vi "Insert Walls in Map.vi"(0 "Map":T1, 1 "Grid size":dbl=0.1, 2 "# safety grids":i32, 3 "Walls":cluster{"Y":dbl, "X":dbl}[](array[cluster])) -> (5 "Updated Map":T1)   [LabVIEW 2009]
uses:
  <vilib>/Analysis/Matrix/Datatypes/RealMatrix.ctl
  <vilib>/Analysis/Matrix/NI_Matrix.lvlib
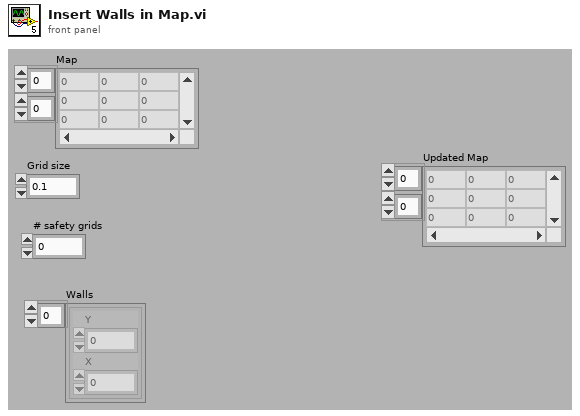
[diagram p1: front panel]
types:
  T1 = typedef "NI_Matrix.lvlib/RealMatrix.ctl" = dbl[][]
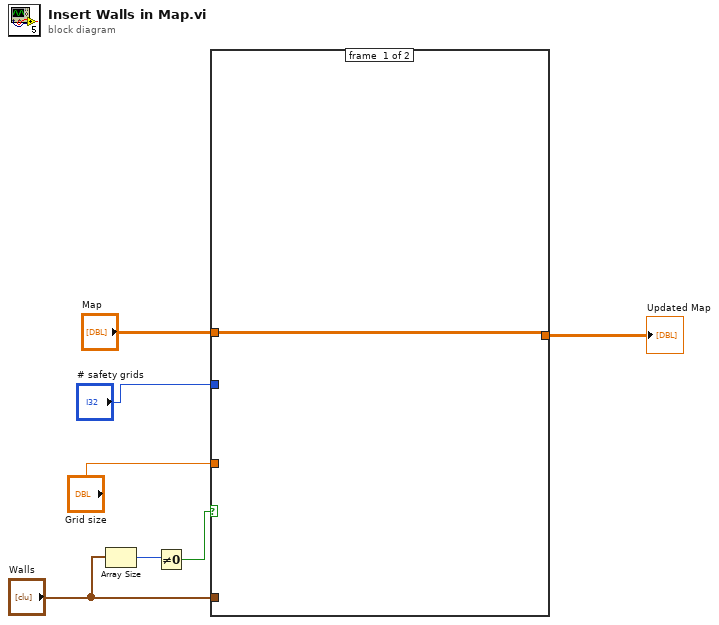
[diagram p0: block diagram]
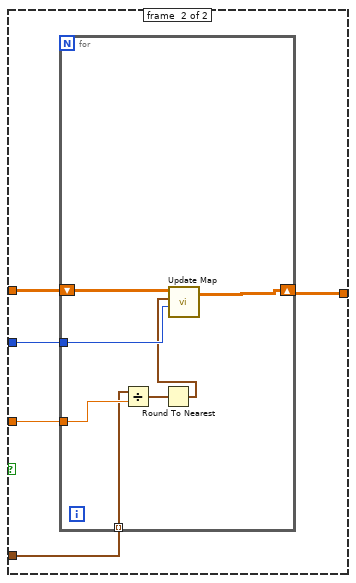
[diagram p2: hidden frame]
diagram:
  n1 = Array Size(array="Walls") -> (size(s)=w3:i32)
  n2 = Not Equal To 0?(x=w3) -> (x != 0?=w2:bool)
  n3 = case shown="True" w2 {
    tunnel: "Walls" -> [_ w13]
    tunnel: "Map" -> [w8 w12]
    tunnel: [w8 w11] -> w6
    tunnel: "# safety grids" -> [_ w10]
    tunnel: "Grid size" -> [_ w9]
    frame #0 {
    }
    frame #1 {
      n4 = for {
        tunnel: w13 -> [w16] mode=indexing
        tunnel: w10 -> [w18]
        shift-right: [w20] -> w11
        shift-left: w12 -> [w19]
        tunnel: w9 -> [w17]
        n5 = Divide(x=w16, y=w17) -> (x/y=w15:cluster{"Y":dbl, "X":dbl})
        n6 = Round To Nearest(number=w15) -> (nearest integer value=w14:cluster{"Y":dbl, "X":dbl})
        n7 = call "Update Map.vi"("# safety grids"=w18, "Point"=w14, "Map"=w19) -> ("Updated Map"=w20:T1)  [unwired: 2 in]
      }
    }
  }
  "Updated Map" <- w6
